vi "Get Response Fit.vi"(8 "error in (no error)":errorcluster, 11 "Halfwave Sinusoidal Fit in":refnum<class "Halfwave Sinusoidal Fit.lvclass">) -> (0 "error out":errorcluster, 2 "Fit out":dbl[](array[numeric]), 3 "Halfwave Sinusoidal Fit out":refnum<class "Halfwave Sinusoidal Fit.lvclass">)   [LabVIEW 2016, in "Halfwave Sinusoidal Fit.lvclass"]
uses:
  Halfwave Sinusoidal Fit.lvclass
  Sinusoidal Fit.lvclass
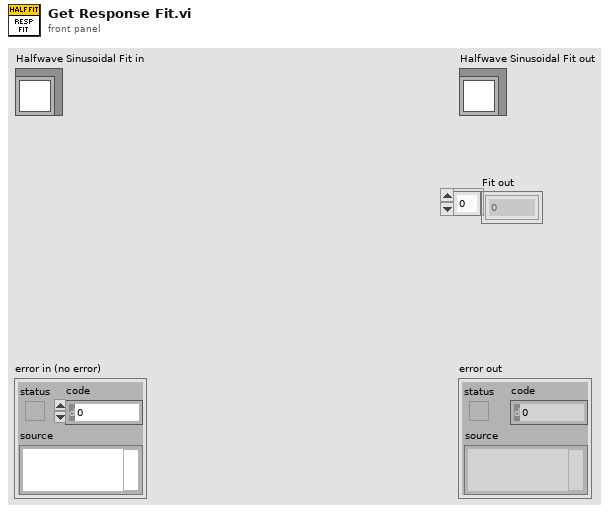
[diagram p1: front panel]
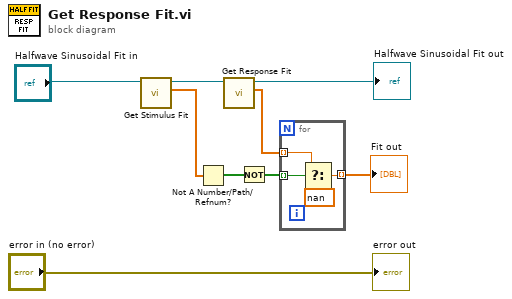
[diagram p0: block diagram]
diagram:
  n1 = call-dynamic "Get Stimulus Fit.vi"("Halfwave Sinusoidal Fit in"="Halfwave Sinusoidal Fit in") -> ("Fit out"=w3:dbl[], "Halfwave Sinusoidal Fit out"=w4:refnum<class "Halfwave Sinusoidal Fit.lvclass">)  [unwired: 8 in, 1 out]
  n2 = Not A Number/Path/Refnum?(number/path/refnum=w3) -> (NaN/Path/Refnum?=w6:bool[])
  n3 = call-parent "Get Response Fit.vi"("Sinusoidal Fit in"=w4) -> ("Fit out"=w1:dbl[], "Sinusoidal Fit out"=→"Halfwave Sinusoidal Fit out":refnum<class "Halfwave Sinusoidal Fit.lvclass">)  [unwired: 8 in, 1 out]
  n4 = Not(x=w6) -> (.not. x?=w7:bool[])
  n5 = for {
    tunnel: w7 -> [w10] mode=indexing
    tunnel: w1 -> [w13] mode=indexing
    tunnel: [w11] -> w8 mode=indexing
    n6 = Select(t=w13, s=w10, f=nan) -> (s? t:f=w11:dbl)
  }
  "Fit out" <- w8
  "error out" <- "error in (no error)"
